vi "PH_Sound.panel.vi"(0 "object ref":refnum<vi>, 5 "error in (no error)":errorcluster) -> (19 "error out":errorcluster)   [LabVIEW 2014, in "PH_Sound.lvlib"]
doc: "By this VI a ross relais can be monitored and switched. \n\nThe indicators \"CLOSED\", \"OPEN\" and \"SWITCH STATE\" show the value of the Beckhoff-Tag: blue indicates bad tag status reference problems, darkgreen false and lightgreen on. If everything is working fine, \"CLOSED\" and \"SWITCH STATE\" should show the same value, while \"OPEN\" has the opposite value. \n\nThe oval button switches the ross relais. It should be in the same state as the \"SWITCH STATE\" indicator. \n\n\"EXIT\" closes the front panel (GUI), while \"Delete Instance\" disconnects and removes the instance from the PCS.\n\nThis VI has no machine safety relevant logig: there is neither a check of internal conclict nor with other objects, for example conflict with other ross relais. Therefore it must be handled with care and should be operated by well educated operators only. It is forseen exclusively for direct operating and testing of the system. \n\nLicense Agreement for this software:\n\nCopyright (C)\nGesellschaft für Schwerionenforschung, GSI\nPlanckstr. 1\n64291 Darmstadt\nGermany\n\nContact: D.Beck@gsi.de \n\nThis program is free software; you can redistribute it and/or modify it under the terms of the GNU General Public License as published by the Free Software Foundation; either version 2 of the license, or (at your option) any later version.\n\nThis program is distributed in the hope that it will be useful, but WITHOUT ANYW ARRANTY; without even the implied warranty of MERCHANTABILITY or FITNESS FOR A PARTICULAR PURPOSE. See the GNU General License for more details (http://www.gnu.org).\n\nGesellschaft für Schwerionenforschung, GSI\nPlanckstr. 1, 64291 Darmstadt, Germany\nFor all questions and ideas contact: M.Richter@gsi.de, H.Brand@gsi.de or D.Beck@gsi.de.\nLast update: 18-DEC-2002"
uses:
  PH_Sound.lvlib
  PH_Sound.3Oktaves.ctl
  CSCore/CSObj/CSObj.lvlib
  CSCore/CSSystem/CSSystemLib/CSSystemLib.lvlib
  PH_Common/PH_Common.lvlib
  PH_Class/PH_Class.lvlib
panel:
  out "Device error":errorcluster
  in  "Timing 3":bool
  in  "Timing 2":bool
  in  "Timing 1":bool caption="Timings"
  out "Emergency Off":bool
  out "Countdown Running":bool
  out "PreAmp-Freigabe":bool
  out "Laserfreigabe":bool
  in  "Countdown Running aus":bool
  in  "Counddown Running ein":bool
  in  "PreAmp-Freigabe aus":bool
  in  "PreAmp-Freigabe ein":bool
  in  "Laserfreigabe aus":bool
  in  "Laserfreigabe ein":bool
  in  "Alarmtest":bool caption="Alarm"
  in  "3 Octaves":T1=130.8 items=["c"=130.8, "cis"=138.6, "d"=146.8, "es"=155.6, "e"=164.8, "f"=174.6, "fis"=185.0, "g"=196.0, "as"=207.6, "a"=220.0, "b"=233.1, "h"=246.9, "c'"=261.6, "cis'"=277.2, "d'"=293.7, "es'"=311.1, "e'"=329.6, "f'"=349.2, "fis'"=370.0, "g'"=392.0, "as'"=415.3, "a'"=440.0, "b'"=466.2, "h'"=493.9, "c''"=523.3, "cis''"=554.4, "d''"=587.3, "es''"=622.3, "e''"=659.3, "f''"=689.5, "fis''"=740.0, "g''"=784.0, "as''"=830.6, "a''"=880.0, "b''"=932.3, "h''"=987.8, "c'''"=1047.0]
  in  "b":bool
  in  "as":bool
  in  "fis":bool
  in  "es":bool
  in  "cis":bool
  in  "h":bool
  in  "a":bool
  in  "g":bool
  in  "f":bool
  in  "e":bool
  in  "d":bool
  in  "c":bool
  in  "b''":bool
  in  "as''":bool
  in  "fis''":bool
  in  "es''":bool
  in  "cis''":bool
  in  "h''":bool
  in  "a''":bool
  in  "g''":bool
  in  "f''":bool
  in  "e''":bool
  in  "d''":bool
  in  "c''":bool
  in  "c'''":bool
  in  "b'":bool
  in  "as'":bool
  in  "fis'":bool
  in  "es'":bool
  in  "cis'":bool
  in  "h'":bool
  in  "a'":bool
  in  "g'":bool
  in  "f'":bool
  in  "e'":bool
  in  "d'":bool
  in  "c'":bool
  in  "Delete":bool
  in  "Exit":bool
  # "PCS"
  # "3.40"
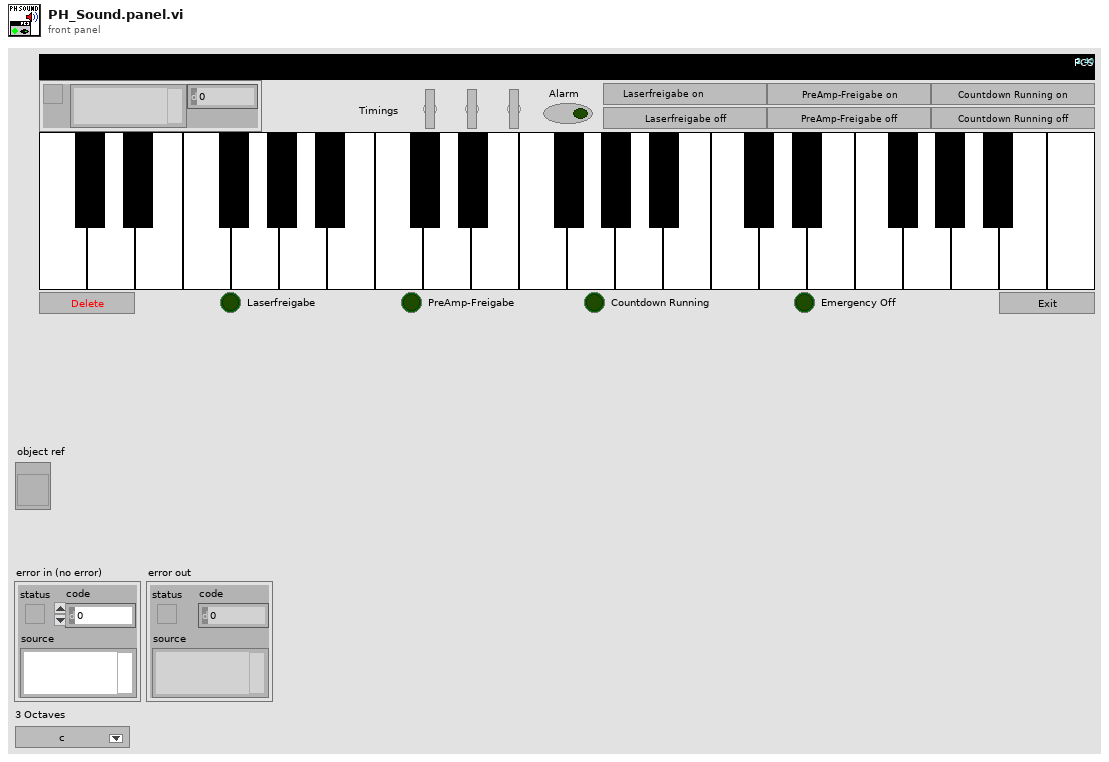
[diagram p1: front panel]
types:
  T1 = typedef "PH_Sound.lvlib/PH_Sound.3Oktaves.ctl" = dbl
  T2 = typedef "LVStringsAndValuesArrayTypeDef_DBL.ctl" = cluster{"String":string, "Value":dbl}[]
  T3 = typedef "PH_Sound.lvlib/PH_Sound.i attribute.ctl" = cluster{"GUI Refs":cluster{"Exit":refnum<vi>, "Laserfreigabe":refnum<vi>, "PreAmp-Freigabe":refnum<vi>, "Countdown Running":refnum<vi>, "Emergency Off":refnum<vi>, "Device Error":refnum<vi>}, "Testalarm on":bool, "State":cluster{"Laser Class 4":bool, "PreAmp Running":bool, "Countdown Running":bool, "Emergency Off":bool}, "Starting Time":timestamp}
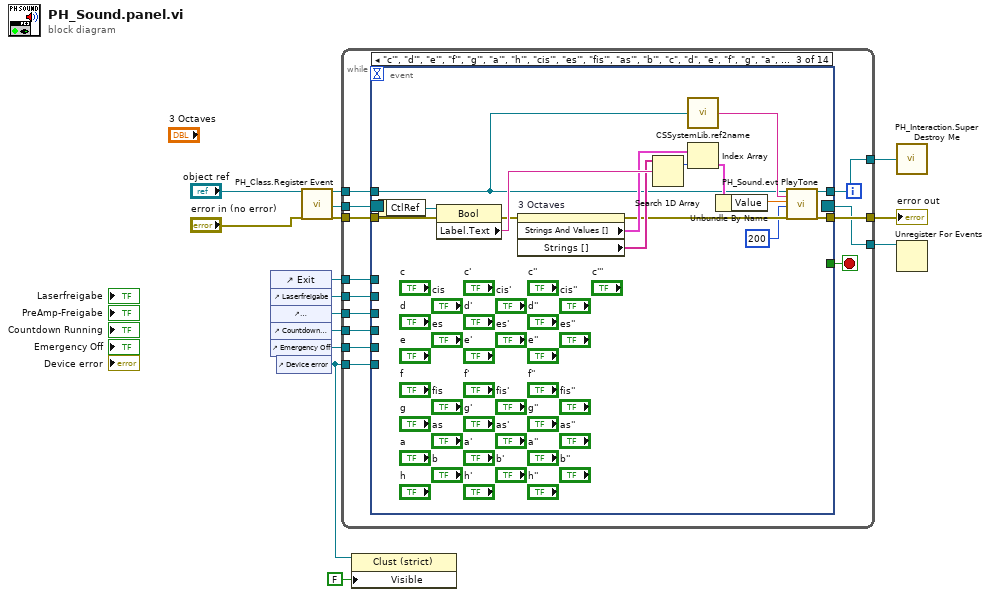
[diagram p0: block diagram]
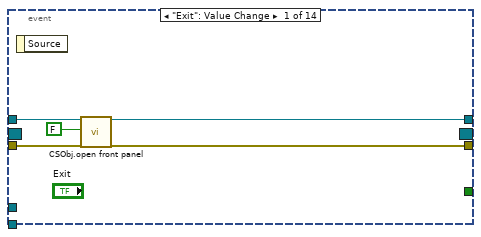
[diagram p2: hidden frame]
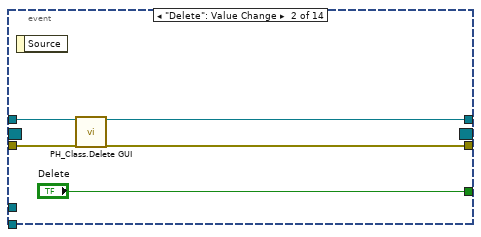
[diagram p3: hidden frame]
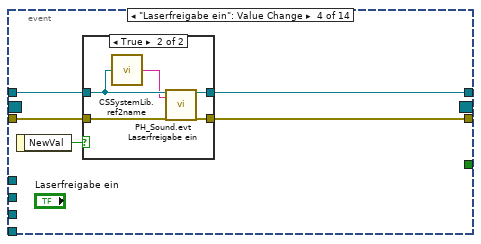
[diagram p4: hidden frame]
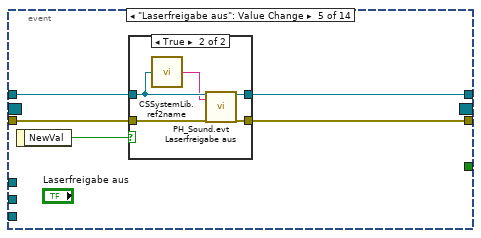
[diagram p6: hidden frame]
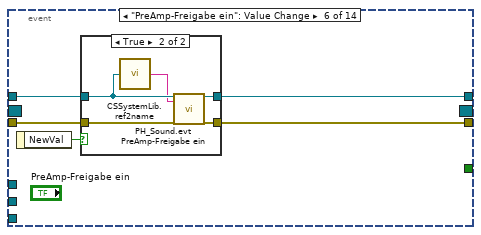
[diagram p8: hidden frame]
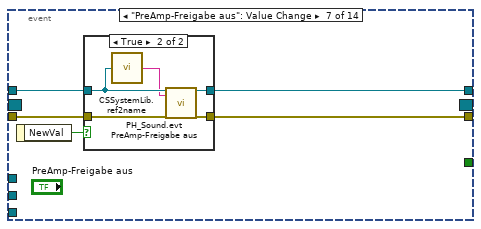
[diagram p10: hidden frame]
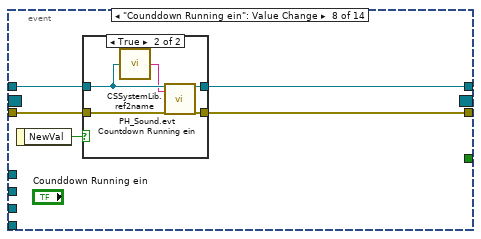
[diagram p12: hidden frame]
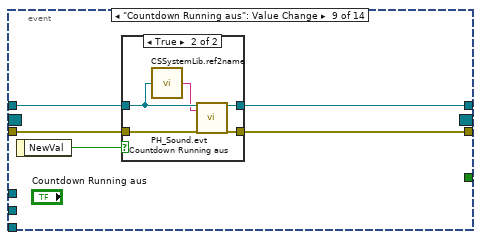
[diagram p14: hidden frame]
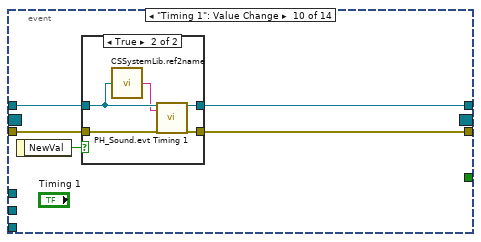
[diagram p16: hidden frame]
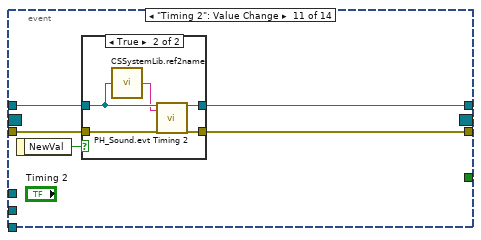
[diagram p18: hidden frame]
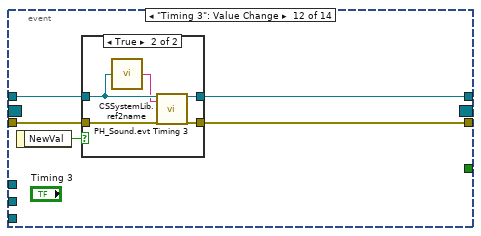
[diagram p20: hidden frame]
diagram:
  n1 = control-ref of="Exit"() -> (w9:refnum<vi>)
  n2 = control-ref of="Laserfreigabe"() -> (w8:refnum<vi>)
  n3 = control-ref of="PreAmp-Freigabe"() -> (w7:refnum<vi>)
  n4 = control-ref of="Countdown Running"() -> (w6:refnum<vi>)
  n5 = control-ref of="Emergency Off"() -> (w5:refnum<vi>)
  n6 = control-ref of="Device error"() -> (w2:refnum<vi>)
  n7 = call "PH_Class.Register Event.vi"("i ref in"="object ref", "error in (no error)"="error in (no error)") -> ("i ref out"=w13:refnum<vi>, "Event Registration Refnum"=w11:refnum<event-registration>, "error out"=w12:errorcluster)  [unwired: 15 in]
  n8 = while {
    tunnel: w13 -> [w25]
    tunnel: [w24] -> w15
    tunnel: w12 -> [w27]
    tunnel: [w26] -> w14
    tunnel: w11 -> [w23]
    tunnel: [w22] -> w10
    tunnel: w9 -> [w21]
    tunnel: w8 -> [w20]
    tunnel: w7 -> [w19]
    tunnel: w6 -> [w18]
    tunnel: w5 -> [w17]
    tunnel: w2 -> [w16]
    stop <- w28 stop-if-true
    n9 = event shown="[2] \"c'\", \"d'\", \"e'\", \"f'\", \"g'\", \"a'\", \"h'\", \"cis'\", \"es'\", \"fis'\", \"as'\", \"b'\", \"c\", \"d\", \"e\", \"f\", \"g\", \"a\", \"h\", \"cis\", \"es\", \"fis\", \"as\", \"b\", \"c''\", \"d''\", \"e''\", \"f''\", \"g''\", \"a''\", \"h''\", \"c'''\", \"cis''\", \"es''\", \"fis''\", \"as''\", \"b''\": Value Change" {
      selector: w23 -> [_ _ _ _ _ _ _ _ _ _ _ _ _ _]
      dyn-events: [_ _ _ _ _ _ _ _ _ _ _ _ _ _] -> w22
      timeout: _ -> [_ _ _ _ _ _ _ _ _ _ _ _ _ _]
      tunnel: [_ "Delete" _ _ _ _ _ _ _ _ _ _ _ _] -> w28
      tunnel: w25 -> [w33 w37 w40 w55 w67 w79 w91 w103 w115 w127 w139 w151 w164 w178]
      tunnel: w27 -> [w31 w36 w49 w58 w70 w82 w94 w106 w118 w130 w142 w154 w167 w177]
      tunnel: [w30 w35 w53 w56 w68 w80 w92 w104 w116 w128 w140 w152 w165 w179] -> w26
      tunnel: [w29 w34 w52 w57 w69 w81 w93 w105 w117 w129 w141 w153 w166 w180] -> w24
      tunnel: w21 -> [_ _ _ _ _ _ _ _ _ _ _ _ _ w173]
      tunnel: w20 -> [_ _ _ _ _ _ _ _ _ _ _ _ _ w172]
      tunnel: w19 -> [_ _ _ _ _ _ _ _ _ _ _ _ _ w171]
      tunnel: w18 -> [_ _ _ _ _ _ _ _ _ _ _ _ _ w170]
      tunnel: w17 -> [_ _ _ _ _ _ _ _ _ _ _ _ _ w169]
      tunnel: w16 -> [_ _ _ _ _ _ _ _ _ _ _ _ _ w168]
      event "Exit": Value Change {
        n10 = event-data() -> ()  [unwired: 1 in, 1 out]
        n11 = call "CSObj.open front panel.vi"("i ref in"=w33, "frontPanelOpen"=FALSE ("front panel open"), "error in (no error)"=w31) -> ("i ref out"=w29:refnum<vi>, "error out"=w30:errorcluster)  [unwired: 15 in]
      }
      event "Delete": Value Change {
        n12 = event-data() -> ()  [unwired: 1 in, 1 out]
        n13 = call "PH_Class.Delete GUI.vi"("VI in"=w37, "error in (no error)"=w36) -> ("VI out"=w34:refnum<vi>, "error out"=w35:errorcluster)  [unwired: 16 in]
      }
      event "c'", "d'", "e'", "f'", "g'", "a'", "h'", "cis'", "es'", "fis'", "as'", "b'", "c", "d", "e", "f", "g", "a", "h", "cis", "es", "fis", "as", "b", "c''", "d''", "e''", "f''", "g''", "a''", "h''", "c'''", "cis''", "es''", "fis''", "as''", "b''": Value Change {
        n14 = event-data() -> ("CtlRef"=w50:refnum<vi>)  [unwired: 1 in]
        n15 = property class="Bool"(reference=w50, error in=w49) -> (error out=w43:errorcluster, "Label.Text"=w48:string)  [unwired: 1 out]
        n16 = property on="3 Octaves" class="Ring (strict)"(error in=w43) -> (error out=w42:errorcluster, "Strings And Values []"=w46:T2, "Strings []"=w47:string[])  [unwired: 1 in, 1 out]
        n17 = Search 1D Array(1D array=w47, element=w48) -> (index of element=w45:i32)  [unwired: 1 in]
        n18 = call "CSSystemLib.ref2name.vi"("obj refnum"=w40) -> ("name"=w51:string)
        n19 = Index Array(array=w46, index=w45) -> (element=w44:cluster{"String":string, "Value":dbl})
        n20 = Unbundle By Name(w44) -> ("Value"=w41:dbl)
        n21 = call "PH_Sound.evt PlayTone .vi"("i ref in"=w40, "Instance"=w51, "Tone"=w41, "Legth [ms]"=200, "error in (no error)"=w42) -> ("i ref out"=w52:refnum<vi>, "error out"=w53:errorcluster)  [unwired: 13 in]
      }
      event "Laserfreigabe ein": Value Change {
        n22 = event-data() -> ("NewVal"=w54:bool)  [unwired: 1 in]
        n23 = case shown="True" w54 {
          tunnel: w58 -> [w59 w65]
          tunnel: [w60 w64] -> w57
          tunnel: [w59 w63] -> w56
          tunnel: w55 -> [w60 w62]
          frame False {
          }
          frame True {
            n24 = call "CSSystemLib.ref2name.vi"("obj refnum"=w62) -> ("name"=w61:string)
            n25 = call "PH_Sound.evt Laserfreigabe ein.vi"("i ref in"=w62, "Instance"=w61, "error in (no error)"=w65) -> ("i ref out"=w64:refnum<vi>, "error out"=w63:errorcluster)  [unwired: 15 in]
          }
        }
      }
      event "Laserfreigabe aus": Value Change {
        n26 = event-data() -> ("NewVal"=w66:bool)  [unwired: 1 in]
        n27 = case shown="True" w66 {
          tunnel: w70 -> [w71 w77]
          tunnel: [w72 w76] -> w69
          tunnel: [w71 w75] -> w68
          tunnel: w67 -> [w72 w74]
          frame False {
          }
          frame True {
            n28 = call "CSSystemLib.ref2name.vi"("obj refnum"=w74) -> ("name"=w73:string)
            n29 = call "PH_Sound.evt Laserfreigabe aus.vi"("i ref in"=w74, "Instance"=w73, "error in (no error)"=w77) -> ("i ref out"=w76:refnum<vi>, "error out"=w75:errorcluster)  [unwired: 15 in]
          }
        }
      }
      event "PreAmp-Freigabe ein": Value Change {
        n30 = event-data() -> ("NewVal"=w78:bool)  [unwired: 1 in]
        n31 = case shown="True" w78 {
          tunnel: w82 -> [w83 w89]
          tunnel: [w84 w88] -> w81
          tunnel: [w83 w87] -> w80
          tunnel: w79 -> [w84 w86]
          frame False {
          }
          frame True {
            n32 = call "CSSystemLib.ref2name.vi"("obj refnum"=w86) -> ("name"=w85:string)
            n33 = call "PH_Sound.evt PreAmp-Freigabe ein.vi"("i ref in"=w86, "Instance"=w85, "error in (no error)"=w89) -> ("i ref out"=w88:refnum<vi>, "error out"=w87:errorcluster)  [unwired: 15 in]
          }
        }
      }
      event "PreAmp-Freigabe aus": Value Change {
        n34 = event-data() -> ("NewVal"=w90:bool)  [unwired: 1 in]
        n35 = case shown="True" w90 {
          tunnel: w94 -> [w95 w101]
          tunnel: [w96 w100] -> w93
          tunnel: [w95 w99] -> w92
          tunnel: w91 -> [w96 w98]
          frame False {
          }
          frame True {
            n36 = call "CSSystemLib.ref2name.vi"("obj refnum"=w98) -> ("name"=w97:string)
            n37 = call "PH_Sound.evt PreAmp-Freigabe aus.vi"("i ref in"=w98, "Instance"=w97, "error in (no error)"=w101) -> ("i ref out"=w100:refnum<vi>, "error out"=w99:errorcluster)  [unwired: 15 in]
          }
        }
      }
      event "Counddown Running ein": Value Change {
        n38 = event-data() -> ("NewVal"=w102:bool)  [unwired: 1 in]
        n39 = case shown="True" w102 {
          tunnel: w106 -> [w107 w113]
          tunnel: [w108 w112] -> w105
          tunnel: [w107 w111] -> w104
          tunnel: w103 -> [w108 w110]
          frame False {
          }
          frame True {
            n40 = call "CSSystemLib.ref2name.vi"("obj refnum"=w110) -> ("name"=w109:string)
            n41 = call "PH_Sound.evt Countdown Running ein.vi"("i ref in"=w110, "Instance"=w109, "error in (no error)"=w113) -> ("i ref out"=w112:refnum<vi>, "error out"=w111:errorcluster)  [unwired: 15 in]
          }
        }
      }
      event "Countdown Running aus": Value Change {
        n42 = event-data() -> ("NewVal"=w114:bool)  [unwired: 1 in]
        n43 = case shown="True" w114 {
          tunnel: w118 -> [w119 w125]
          tunnel: [w120 w124] -> w117
          tunnel: [w119 w123] -> w116
          tunnel: w115 -> [w120 w122]
          frame False {
          }
          frame True {
            n44 = call "CSSystemLib.ref2name.vi"("obj refnum"=w122) -> ("name"=w121:string)
            n45 = call "PH_Sound.evt Countdown Running aus.vi"("i ref in"=w122, "Instance"=w121, "error in (no error)"=w125) -> ("i ref out"=w124:refnum<vi>, "error out"=w123:errorcluster)  [unwired: 15 in]
          }
        }
      }
      event "Timing 1": Value Change {
        n46 = event-data() -> ("NewVal"=w126:bool)  [unwired: 1 in]
        n47 = case shown="True" w126 {
          tunnel: w130 -> [w131 w137]
          tunnel: [w132 w136] -> w129
          tunnel: [w131 w135] -> w128
          tunnel: w127 -> [w132 w134]
          frame False {
          }
          frame True {
            n48 = call "CSSystemLib.ref2name.vi"("obj refnum"=w134) -> ("name"=w133:string)
            n49 = call "PH_Sound.evt Timing 1.vi"("i ref in"=w134, "Instance"=w133, "error in (no error)"=w137) -> ("i ref out"=w136:refnum<vi>, "error out"=w135:errorcluster)  [unwired: 15 in]
          }
        }
      }
      event "Timing 2": Value Change {
        n50 = event-data() -> ("NewVal"=w138:bool)  [unwired: 1 in]
        n51 = case shown="True" w138 {
          tunnel: w142 -> [w143 w149]
          tunnel: [w144 w148] -> w141
          tunnel: [w143 w147] -> w140
          tunnel: w139 -> [w144 w146]
          frame False {
          }
          frame True {
            n52 = call "CSSystemLib.ref2name.vi"("obj refnum"=w146) -> ("name"=w145:string)
            n53 = call "PH_Sound.evt Timing 2.vi"("i ref in"=w146, "Instance"=w145, "error in (no error)"=w149) -> ("i ref out"=w148:refnum<vi>, "error out"=w147:errorcluster)  [unwired: 15 in]
          }
        }
      }
      event "Timing 3": Value Change {
        n54 = event-data() -> ("NewVal"=w150:bool)  [unwired: 1 in]
        n55 = case shown="True" w150 {
          tunnel: w154 -> [w155 w161]
          tunnel: [w156 w160] -> w153
          tunnel: [w155 w159] -> w152
          tunnel: w151 -> [w156 w158]
          frame False {
          }
          frame True {
            n56 = call "CSSystemLib.ref2name.vi"("obj refnum"=w158) -> ("name"=w157:string)
            n57 = call "PH_Sound.evt Timing 3.vi"("i ref in"=w158, "Instance"=w157, "error in (no error)"=w161) -> ("i ref out"=w160:refnum<vi>, "error out"=w159:errorcluster)  [unwired: 15 in]
          }
        }
      }
      event "Alarmtest": Value Change {
        n58 = event-data() -> ("NewVal"=w162:bool)  [unwired: 1 in]
        n59 = call "CSSystemLib.ref2name.vi"("obj refnum"=w164) -> ("name"=w163:string)
        n60 = call "PH_Sound.evt Probealarm.vi"("i ref in"=w164, "Instance"=w163, "Testalarm on"=w162, "error in (no error)"=w167) -> ("i ref out"=w166:refnum<vi>, "error out"=w165:errorcluster)  [unwired: 14 in]
      }
      event User Event {
        n61 = event-data() -> ("Class"=w174:string)  [unwired: 1 in]
        n62 = case shown="\"PH_Sound\"" w174 {
          tunnel: w178 -> [w182 w192]
          tunnel: w177 -> [w181 w191]
          tunnel: [w181 w190] -> w176
          tunnel: [w182 w189] -> w175
          tunnel: w173 -> [_ w188]
          tunnel: w172 -> [_ w187]
          tunnel: w171 -> [_ w186]
          tunnel: w170 -> [_ w185]
          tunnel: w169 -> [_ w184]
          tunnel: w168 -> [_ w183]
          frame Default {
          }
          frame "PH_Sound" {
            n63 = call "PH_Sound.get data to modify.vi"("i ref in"=w192, "ms timeout (10000)"=-1, "error in (no error)"=w191) -> ("i ref out"=w193:refnum<vi>, "i attribute"=w196:T3, "error out"=w194:errorcluster)  [unwired: 13 in, 1 out]
            n64 = Bundle By Name(cluster=w196, "GUI Refs.Exit"=w188, "GUI Refs.Laserfreigabe"=w187, "GUI Refs.PreAmp-Freigabe"=w186, "GUI Refs.Countdown Running"=w185, "GUI Refs.Emergency Off"=w184, "GUI Refs.Device Error"=w183) -> (w197:T3)
            n65 = call "PH_Sound.set modified data.vi"("i ref in"=w193, "i attribute"=w197, "error in (no error)"=w194) -> ("i ref out"=w189:refnum<vi>, "error out"=w190:errorcluster)  [unwired: 15 in]
          }
        }
        n66 = call "PH_Class.set GUI Refs stored Occurence.vi"("i ref in"=w175, "error in (no error)"=w176) -> ("i ref out"=w180:refnum<vi>, "error out"=w179:errorcluster)  [unwired: 16 in]
      }
    }
  }
  "error out" <- w14
  n67 = property class="Clust (strict)"(reference=w2, "Visible"=FALSE) -> ()  [unwired: 1 in, 2 out]
  n68 = call "PH_Interaction.Super Destroy Me.vi"("i ref out"=w15) -> ()
  n69 = Unregister For Events(event registration refnum=w10) -> ()  [unwired: 1 in, 1 out]
